vi "slowscan_graph.vi"(4 "y min":dbl, 6 "y pts flyback":i32, 7 "y pixels":i32, 8 "x pts flyback":i32, 9 "Samples to Average":i32, 10 "y max":dbl, 11 "x pixels":i32) -> (3 "Array out":dbl[](array[numeric]))   [LabVIEW 2012]
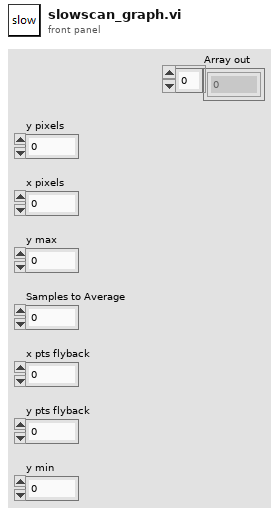
[diagram p1: front panel]
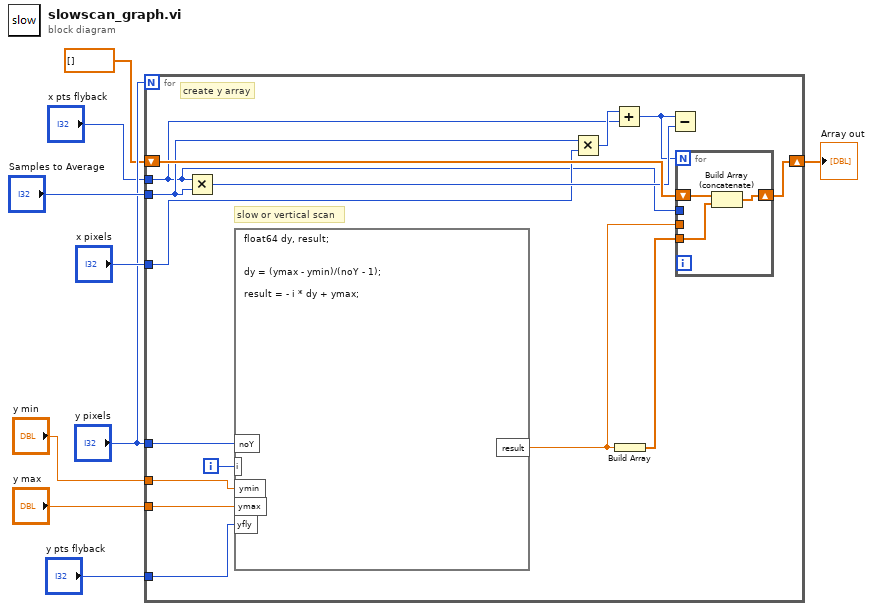
[diagram p0: block diagram]
diagram:
  n1 = for {
    N: "y pixels" -> [_]
    tunnel: "y pixels" -> [w21]
    tunnel: "y min" -> [w19]
    tunnel: "y max" -> [w23]
    shift-right: [w13] -> w5
    shift-left: dbl[] [] -> [w22]
    tunnel: "x pixels" -> [w16]
    tunnel: "x pts flyback" -> [w11]
    tunnel: "y pts flyback" -> [w20]
    tunnel: "Samples to Average" -> [w17]
    i -> [w24]
    # "slow or vertical scan"
    # "create y array"
    n2 = Multiply(x=w11, y=w17) -> (x*y=w18:i32)
    n3 = formula code="float64 dy, result;\n\n\ndy = (ymax - ymin)/(noY - 1);\n\nresult = - i * dy + ymax;"("i"=w24, "ymin"=w19, "ymax"=w23, "noY"=w21, "yfly"=w20) -> ("result"=w14:dbl)
    n4 = Multiply(x=w17, y=w16) -> (x*y=w12:i32)
    n5 = Add(x=w12, y=w11) -> (x+y=w10:i32)
    n6 = Build Array(w14) -> (w15:dbl[])
    n7 = Subtract(x=w10, y=w18) -> ()  [unwired: 1 out]
    n8 = for {
      N: w10 -> [_]
      tunnel: w15 -> [w26]
      shift-right: [w25] -> w13
      shift-left: w22 -> [w27]
      tunnel: w14 -> [_]
      tunnel: w11 -> [_]
      n9 = Build Array (concatenate)(w27, w26) -> (w25:dbl[])
    }
  }
  "Array out" <- w5
